vi "Dequeue Published Result.vi"(8 "error in (no error)":errorcluster, 9 "timeout in ms (-1)":i32, 11 "Mock Result Observer In":refnum<class "Mock Result Observer.lvclass">) -> (0 "error out":errorcluster, 1 "timed out?":bool, 2 "Result":T1={"Name"="", "Message"="", "Description"="", "Status"=enum."Passed", "Result Type"=enum."Case", "Execution Time"=0.0}, 3 "Mock Result Observer Out":refnum<class "Mock Result Observer.lvclass">)   [LabVIEW 2020, in "Mock Result Observer.lvclass"]
uses:
  Mock Result Observer.lvclass
  Core/Result/Result.ctl
  Core/Result/Status.ctl
  Core/Result/Type.ctl
  Mock Result Observer.lvclass/Mock Result Observer.ctl
  Core/Result/Result.lvlib
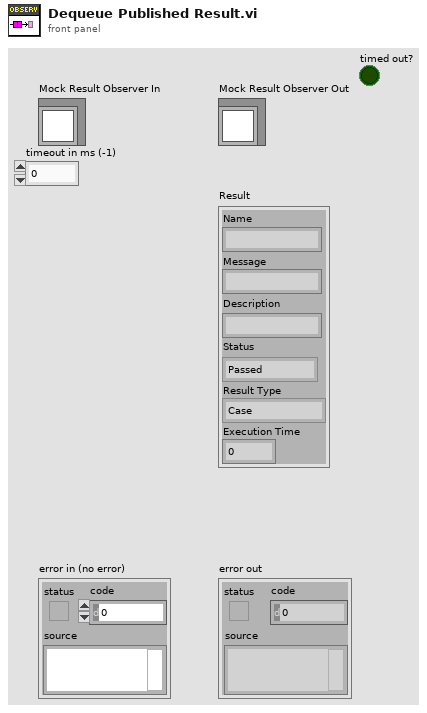
[diagram p1: front panel]
types:
  T1 = typedef "Result.lvlib/Result.ctl" = cluster{"Name":string, "Message":string, "Description":string, "Status":T2, "Result Type":T3, "Execution Time":dbl}
  T2 = typedef "Result.lvlib/Status.ctl" = enum16{"", "Passed", "Failed", "Error", "Skipped", "Setup Error", "Broken", "Teardown Error"}
  T3 = typedef "Result.lvlib/Type.ctl" = enum16{"Method", "Case", "Suite", "Pass", "Fail", "Skip", "Pass if", "Fail if", "Pass if Error", "Fail if Error", "Pass if Equal", "Fail if Equal"}
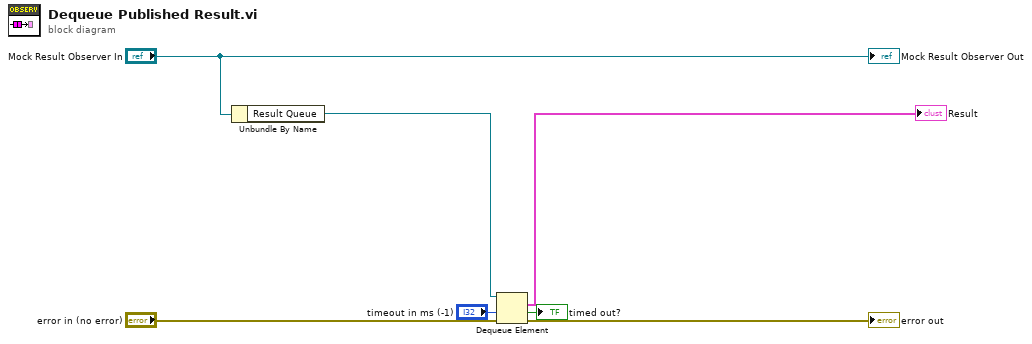
[diagram p0: block diagram]
diagram:
  n1 = Unbundle By Name("Mock Result Observer In") -> ("Result Queue"=w4:refnum<queue>)
  n2 = Dequeue Element(queue=w4, timeout in ms (-1)="timeout in ms (-1)", error in (no error)="error in (no error)") -> (element=→"Result":T1, timed out?=→"timed out?":bool, error out=→"error out":errorcluster)  [unwired: 1 out]
  "Mock Result Observer Out" <- "Mock Result Observer In"
